vi "RSZVB Insert New Segment.vi"(0 "VISA session":refnum<visa-resource-name>, 1 "Channel (1)":i32=1, 2 "Segment (1)":i32=1, 3 "Start Frequency (0.0 Hz)":dbl format="%^.3e", 4 "Stop Frequency (0.0 Hz)":dbl format="%^.3e", 5 "error in (no error)":errorcluster {"code" format="%.0x"}, 6 "Power (0.0 dBm)":dbl format="%^.3e", 7 "Sweep Time Select (0: Time)":i32(ring) items=["Time", "Point Delay"], 8 "Time (21.0 s)":dbl=21.0 format="%^.3e", 9 "Point Delay (0.0 s)":dbl format="%^.3e", 10 "Number Of Points (51)":i32=51, 11 "Meas Bandwidth (10.0e3)":dbl=10000.0 format="%^.3e") -> (14 "dup VISA session":refnum<visa-resource-name>, 19 "error out":errorcluster {"code" format="%.0x"})   [LabVIEW 2011]
doc: "This VI inserts a new sweep segment with specific channel settings. The new segment must not overlap with any of the existing segments.\n\nRemote-control command(s):\n[SENSe<Ch>:]SEGMent<Seg>:INSert\n[SENSe<Ch>:]SEGMent<Seg>:INSert:SELect SWTime | DWELl"
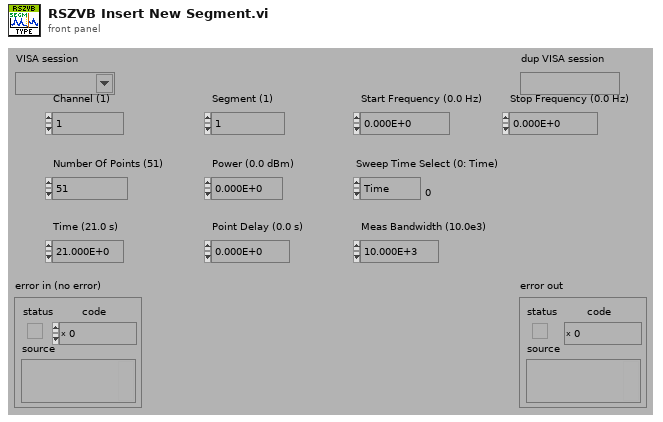
[diagram p1: front panel]
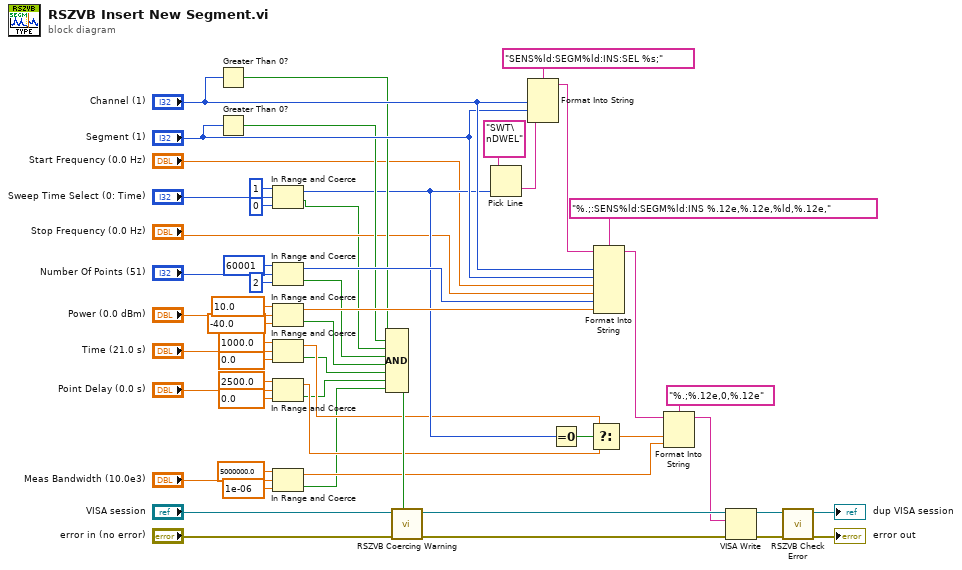
[diagram p0: block diagram]
diagram:
  n1 = Greater Than 0?(x="Channel (1)") -> (x > 0?=w22:bool)
  n2 = Greater Than 0?(x="Segment (1)") -> (x > 0?=w21:bool)
  n3 = In Range and Coerce(upper limit=1, x="Sweep Time Select (0: Time)", lower limit=0) -> (coerced(x)=w14:i32, In Range?=w6:bool)
  n4 = In Range and Coerce(upper limit=60001, x="Number Of Points (51)", lower limit=2) -> (coerced(x)=w24:i32, In Range?=w5:bool)
  n5 = In Range and Coerce(upper limit=10.0, x="Power (0.0 dBm)", lower limit=-40.0) -> (coerced(x)=w23:dbl, In Range?=w4:bool)
  n6 = In Range and Coerce(upper limit=1000.0, x="Time (21.0 s)", lower limit=0.0) -> (coerced(x)=w13:dbl, In Range?=w3:bool)
  n7 = In Range and Coerce(upper limit=2500.0, x="Point Delay (0.0 s)", lower limit=0.0) -> (coerced(x)=w12:dbl, In Range?=w2:bool)
  n8 = In Range and Coerce(upper limit=5000000.0, x="Meas Bandwidth (10.0e3)", lower limit=1e-06) -> (coerced(x)=w9:dbl, In Range?=w1:bool)
  n9 = Compound Arithmetic op=AND(w22, w21, w6, w5, w4, w3, w2, w1) -> (w51:bool)
  n10 = call "RSZVB Coercing Warning.vi"("In Range?"=w51, "error in (no error)"="error in (no error)", "VISA session"="VISA session") -> ("error out"=w54:errorcluster, "dup VISA session"=w55:refnum<visa-resource-name>)  [unwired: 7 in]
  n11 = Pick Line(multi-line string="SWT\nDWEL", line index=w14) -> (output string=w29:string)  [unwired: 1 in]
  n12 = Format Into String(format string="SENS%ld:SEGM%ld:INS:SEL %s;", "Channel (1)", "Segment (1)", w29) -> (resulting string=w27:string)  [unwired: 2 in, 1 out]
  n13 = Equal To 0?(x=w14) -> (x = 0?=w16:bool)
  n14 = Select(t=w13, s=w16, f=w12) -> (s? t:f=w15:dbl)
  n15 = Format Into String(format string="%.;:SENS%ld:SEGM%ld:INS %.12e,%.12e,%ld,%.12e,", initial string=w27, "Channel (1)", "Segment (1)", "Start Frequency (0.0 Hz)", "Stop Frequency (0.0 Hz)", w24, w23) -> (resulting string=w11:string)  [unwired: 1 in, 1 out]
  n16 = Format Into String(format string="%.;%.12e,0,%.12e", initial string=w11, w15, w9) -> (resulting string=w10:string)  [unwired: 1 in, 1 out]
  n17 = VISA Write(VISA resource name=w55, write buffer=w10, error in (no error)=w54) -> (VISA resource name out=w52:refnum<visa-resource-name>, error out=w53:errorcluster)  [unwired: 1 out]
  n18 = call "RSZVB Check Error.vi"("error in (no error)"=w53, "VISA session"=w52) -> ("error out"=→"error out":errorcluster, "dup VISA session"=→"dup VISA session":refnum<visa-resource-name>)  [unwired: 8 in]
